vi "edittest delete step.vi"(8 "error in (no error)":errorcluster, 9 "POST (empty)":T2, 10 "sxSequenceId (\"\")":string, 11 "Connection Refnum":T1) -> (0 "error out":errorcluster, 3 "Connection Refnum":T1)   [LabVIEW 2011]
uses:
  ITK EXT/utils/keyedarr.llb/Keyed Array.ctl
  Summitek EXT/ODBC/SQL Controls/Connection Refnum.ctl
  ITK EXT/utils/strutil.llb/Case Matching.ctl
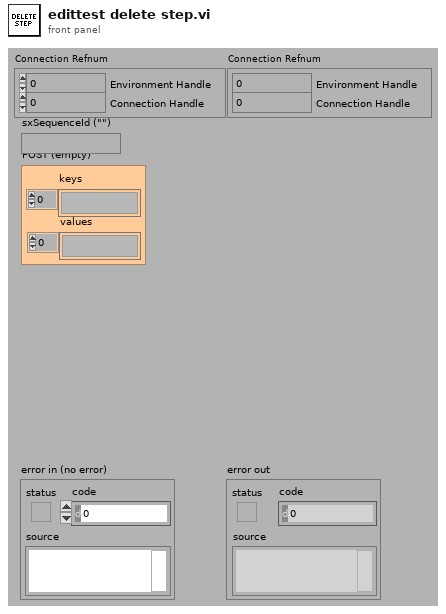
[diagram p1: front panel]
types:
  T1 = typedef "Connection Refnum.ctl" = cluster{"Environment Handle":i32, "Connection Handle":i32}
  T2 = typedef "Keyed Array.ctl" = cluster{"keys":string[], "values":string[]}
  T3 = typedef "Case Matching.ctl" = enum16{"a != A", "a == A", "system"}
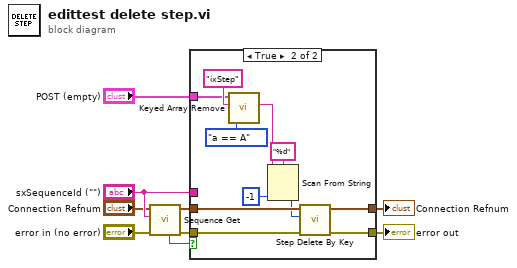
[diagram p0: block diagram]
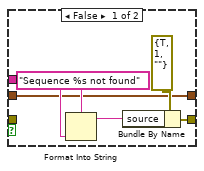
[diagram p2: hidden frame]
diagram:
  n1 = call "Sequence Get.vi"("error in (no error)"="error in (no error)", "sxSequenceId (\"\")"="sxSequenceId (\"\")", "Connection Refnum"="Connection Refnum") -> ("error out"=w6:errorcluster, "Connection Refnum"=w1:T1, "Data Present"=w5:bool)  [unwired: 6 out]
  n2 = case shown="True" w5 {
    tunnel: [w12 w26] -> w9
    tunnel: "POST (empty)" -> [_ w19]
    tunnel: w6 -> [_ w17]
    tunnel: "sxSequenceId (\"\")" -> [w14 _]
    tunnel: [w10 w25] -> w3
    tunnel: w1 -> [w10 w18]
    frame False {
      n3 = Format Into String(format string="Sequence %s not found" ("source"), w14) -> (resulting string=w11:string)  [unwired: 2 in, 1 out]
      n4 = Bundle By Name(cluster=errorcluster {"status"=TRUE, "code"=1, "source"=""} ("error out"), "source"=w11) -> (w12:errorcluster)
    }
    frame True {
      n5 = call "Keyed Array Remove.vi"("case matching (sensitive)"=Case_Matching."a == A", "key"="ixStep", "array in"=w19) -> ("value"=w20:string)  [unwired: 4 out]
      n6 = Scan From String(format string="%d", input string=w20, default 1=-1 ("default value 1")) -> (output 1=w16:i32)  [unwired: 2 in, 3 out]
      n7 = call "Step Delete By Key.vi"("error in (no error)"=w17, "ixStep (0)"=w16, "Connection Refnum"=w18) -> ("error out"=w26:errorcluster, "Connection Refnum"=w25:T1)  [unwired: 7 in]
    }
  }
  "error out" <- w9
  "Connection Refnum" <- w3
